vi "RT_Angular Aceleration in DLR Navigation Reference System(SubVI).vi"(0 "Mco (Nm)":dbl[](array[numeric]), 1 "MFE (Nm)":dbl[](array[numeric]), 2 "MFA (Nm)":dbl[](array[numeric]), 3 "W (rad/s)":dbl[](array[numeric]), 4 "MA_f [Nm]":dbl[](array[numeric]), 5 "MAd [Nm]":dbl[](array[numeric]), 7 "DCM":dbl[][](array[numeric]), 9 "Data":dbl[][](array[numeric]), 11 "i":i32) -> (14 "ang_acc":dbl[](array[numeric]))   [LabVIEW 2017]
uses:
  <vilib>/Analysis/_algsub.llb/Real PseudoInverse Matrix.vi
  <vilib>/Analysis/baseanly.llb/Real A x B.vi
  <vilib>/Analysis/Matrix/Numeric/Conversions/Array To Matrix - RA.vi
  <vilib>/Analysis/Matrix/Numeric/Conversions/Array To Matrix - RA2.vi
  <vilib>/Analysis/Matrix/Numeric/Conversions/Matrix To Array - RM.vi
  <vilib>/Analysis/NI_AALBase.lvlib
  <vilib>/Analysis/Matrix/NI_Matrix.lvlib
  <vilib>/Analysis/NI_AALPro.lvlib
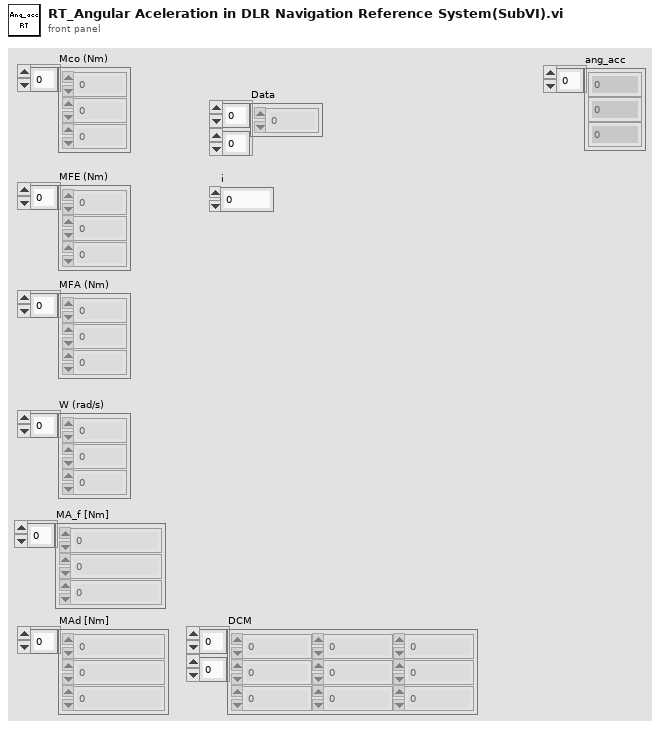
[diagram p1: front panel]
types:
  T1 = typedef "NI_Matrix.lvlib/RealMatrix.ctl" = dbl[][]
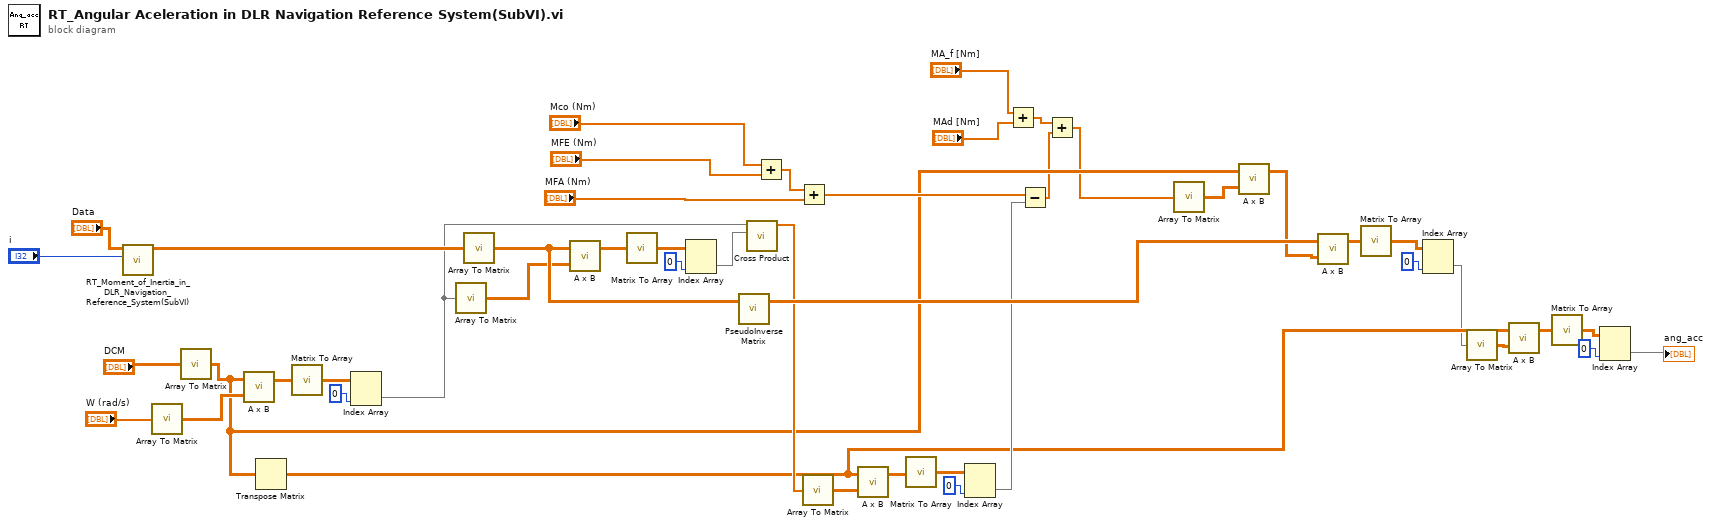
[diagram p0: block diagram]
diagram:
  n1 = call "RT_Moment_of_Inertia_in_DLR_Navigation_Reference_System(SubVI).vi"("i"="i", "Data"="Data") -> ("I (kg.m^2)"=w24:dbl[][])  [unwired: 9 in]
  n2 = call-poly <vilib>:"Array To Matrix.vi"("Real 1D Array"="W (rad/s)") -> ("Real Matrix (Column Vector)"=w29:T1)
  n3 = call-poly <vilib>:"Array To Matrix.vi"("Real 2D Array"="DCM") -> ("Real Matrix"=w16:T1)
  n4 = call-poly <vilib>:"A x B.vi"("B"=w29, "A"=w16) -> ("A x B"=w27:T1)  [unwired: 1 out]
  n5 = Transpose Matrix(1:w16) -> (0:w12:T1)
  n6 = call-poly <vilib>:"Matrix To Array.vi"("Real Matrix"=w27) -> ("Real 2D Array"=w28:dbl[][])
  n7 = Index Array(array=w28, index (col)=0 ("index (row)")) -> (element=w23:dbl[])  [unwired: 1 in]
  n8 = call-poly <vilib>:"Array To Matrix.vi"("Real 1D Array"=w23) -> ("Real Matrix (Column Vector)"=w41:T1)
  n9 = call-poly <vilib>:"Array To Matrix.vi"("Real 2D Array"=w24) -> ("Real Matrix"=w43:T1)
  n10 = call-poly <vilib>:"A x B.vi"("B"=w41, "A"=w43) -> ("A x B"=w39:T1)  [unwired: 1 out]
  n11 = call-poly <vilib>:"Matrix To Array.vi"("Real Matrix"=w39) -> ("Real 2D Array"=w40:dbl[][])
  n12 = Index Array(array=w40, index (col)=0 ("index (row)")) -> (element=w42:dbl[])  [unwired: 1 in]
  n13 = call-poly <vilib>:"PseudoInverse Matrix.vi"("Input Matrix"=w43) -> ("PseudoInverse Matrix"=w44:T1)  [unwired: 1 in, 1 out]
  n14 = call <vilib>:"Cross Product.vi"("B Vector"=w42, "A Vector"=w23) -> ("Cross Product"=w22:dbl[])  [unwired: 8 in, 1 out]
  n15 = Add(x="Mco (Nm)", y="MFE (Nm)") -> (x+y=w34:dbl[])
  n16 = Add(x=w34, y="MFA (Nm)") -> (x+y=w35:dbl[])
  n17 = call-poly <vilib>:"Array To Matrix.vi"("Real 1D Array"=w22) -> ("Real Matrix (Column Vector)"=w21:T1)
  n18 = call-poly <vilib>:"A x B.vi"("B"=w21, "A"=w12) -> ("A x B"=w18:T1)  [unwired: 1 out]
  n19 = call-poly <vilib>:"Matrix To Array.vi"("Real Matrix"=w18) -> ("Real 2D Array"=w19:dbl[][])
  n20 = Index Array(array=w19, index (col)=0 ("index (row)")) -> (element=w17:dbl[])  [unwired: 1 in]
  n21 = Add(x="MA_f [Nm]", y="MAd [Nm]") -> (x+y=w4:dbl[])
  n22 = Subtract(x=w35, y=w17) -> (x-y=w5:dbl[])
  n23 = Add(x=w4, y=w5) -> (x+y=w6:dbl[])
  n24 = call-poly <vilib>:"Array To Matrix.vi"("Real 1D Array"=w6) -> ("Real Matrix (Column Vector)"=w15:T1)
  n25 = call-poly <vilib>:"A x B.vi"("B"=w15, "A"=w16) -> ("A x B"=w14:T1)  [unwired: 1 out]
  n26 = call-poly <vilib>:"A x B.vi"("B"=w14, "A"=w44) -> ("A x B"=w45:T1)  [unwired: 1 out]
  n27 = call-poly <vilib>:"Matrix To Array.vi"("Real Matrix"=w45) -> ("Real 2D Array"=w46:dbl[][])
  n28 = Index Array(array=w46, index (col)=0 ("index (row)")) -> (element=w11:dbl[])  [unwired: 1 in]
  n29 = call-poly <vilib>:"Array To Matrix.vi"("Real 1D Array"=w11) -> ("Real Matrix (Column Vector)"=w10:T1)
  n30 = call-poly <vilib>:"A x B.vi"("B"=w10, "A"=w12) -> ("A x B"=w13:T1)  [unwired: 1 out]
  n31 = call-poly <vilib>:"Matrix To Array.vi"("Real Matrix"=w13) -> ("Real 2D Array"=w8:dbl[][])
  n32 = Index Array(array=w8, index (col)=0 ("index (row)")) -> (element=→"ang_acc":dbl[])  [unwired: 1 in]
